vi "Compression_Simulation_Get POUTs.vi"(7 "PxdB":dbl, 9 "Linear Gain":dbl, 10 "GAINs in":dbl[](array[numeric]), 11 "PINs in":dbl[](array[numeric])) -> (2 "OPxdB":dbl, 3 "POUTs out":dbl[](array[numeric]))   [LabVIEW 2023]
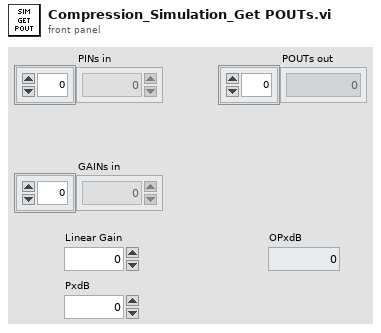
[diagram p1: front panel]
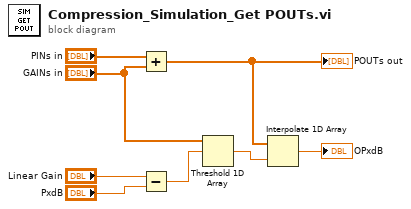
[diagram p0: block diagram]
diagram:
  n1 = Add(x="PINs in", y="GAINs in") -> (x+y=w5:dbl[])
  "POUTs out" <- w5
  n2 = Subtract(x="Linear Gain", y="PxdB") -> (x-y=w7:dbl)
  n3 = Threshold 1D Array(2:w7, 3:"GAINs in") -> (0:w6:dbl)  [unwired: 1 in]
  n4 = Interpolate 1D Array(1:w6, 2:w5) -> (0:→"OPxdB":dbl)
